vi "2_termometro_loop.vi"() -> ()   [LabVIEW 2017]
panel:
  out "Celsius":dbl
  in  "Chave 2":bool
  in  "Chave 1":bool
  out "Waveform Chart":dbl(graph)
  out "Iterações":i32
  out "Kelvin":string
  out "Kelvin":dbl(slide) scale=0.0..500.0 scale format="%.2f"
  out "Fahrenheit":string
  in  "Temperatura":dbl
  out "Fahrenheit":dbl(slide) scale=0.0..250.0 scale format="%.2f"
  # "Kelvin"
  # "Fahrenheit"
  # "Manual"
  # "Automatico"
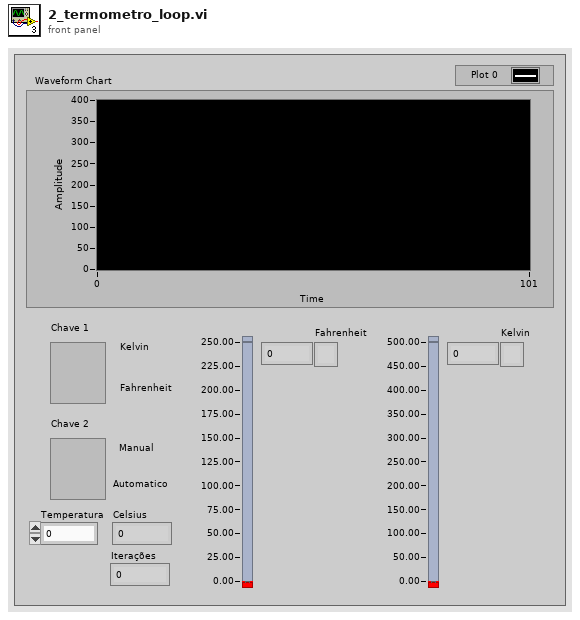
[diagram p1: front panel]
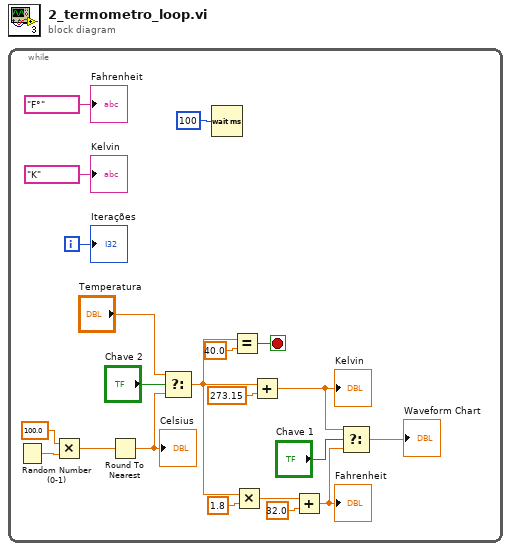
[diagram p0: block diagram]
diagram:
  n1 = while {
    i -> [w15]
    stop <- w9 stop-if-true
    n2 = Random Number (0-1)() -> (number: 0 to 1=w6:dbl)
    n3 = Multiply(x=100.0, y=w6) -> (x*y=w3:dbl)
    n4 = Round To Nearest(number=w3) -> (nearest integer value=w2:dbl)
    "Celsius" <- w2
    n5 = Select(t="Temperatura", s="Chave 2", f=w2) -> (s? t:f=w8:dbl)
    n6 = Wait (ms)(milliseconds to wait=u32 100) -> ()  [unwired: 1 out]
    n7 = Equal?(x=w8, y=40.0) -> (x = y?=w9:bool)
    n8 = Multiply(x=w8, y=1.8) -> (x*y=w20:dbl)
    n9 = Add(x=w8, y=273.15) -> (x+y=w12:dbl)
    "Kelvin" <- w12
    n10 = Add(x=w20, y=32.0) -> (x+y=w11:dbl)
    "Fahrenheit" <- w11
    n11 = Select(t=w12, s="Chave 1", f=w11) -> (s? t:f=→"Waveform Chart":dbl)
    "Fahrenheit" <- "F°"
    "Kelvin" <- "K"
    "Iterações" <- w15
  }
